vi "WSData.vi"() -> ()   [LabVIEW 2019]
panel:
  in  "Logging Interval [s]":dbl=1.0
  in  "DataEU":dbl[](array[numeric]) format="%.2g"
  in  "DataRaw":dbl[](array[numeric]) format="%.2g"
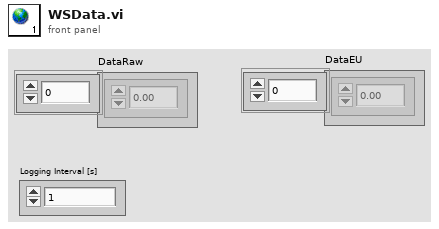
[diagram p1: front panel]
diagram:
